vi "Factory.vi"(8 "error in (no error)":errorcluster, 11 "Measurement Interface in":refnum<class "Measurement Interface.lvclass">=refnum) -> (0 "error out":errorcluster, 3 "Measurement Interface out":refnum<class "Measurement Interface.lvclass">)   [LabVIEW 2016, in "Measurement Interface.lvlib" / "Measurement Interface.lvclass"]
uses:
  Measurement Interface.lvclass
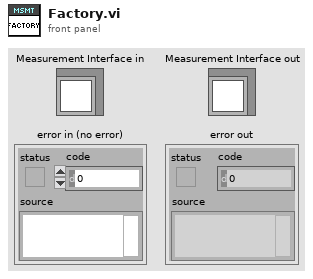
[diagram p1: front panel]
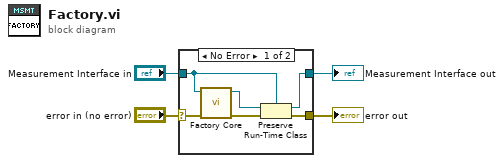
[diagram p0: block diagram]
diagram:
  n1 = case shown="No Error" "error in (no error)" {
    selector: "error in (no error)" -> [w9 w12]
    tunnel: [w8 w12] -> w3
    tunnel: [w6 w11] -> w1
    tunnel: "Measurement Interface in" -> [w5 w11]
    frame No Error {
      n2 = call-dynamic "Factory Core.vi"("error in (no error)"=w9, "Factory Plugin Framework in"=w5) -> ("error out"=w10:errorcluster, "Factory Plugin Framework out"=w7:refnum<class "Measurement Interface.lvclass">)  [unwired: 8 in]
      n3 = Preserve Run-Time Class(object in=w7, error in=w10, 2:w5) -> (object out=w6:refnum<class "Measurement Interface.lvclass">, error out=w8:errorcluster)
    }
    frame Error {
    }
  }
  "error out" <- w3
  "Measurement Interface out" <- w1
